vi "Exercise 3.6.vi"(8 "Focal Length":dbl format="%#_g mm", 9 "Groove Density":dbl format="%#_g grooves/mm", 10 "Requested Wavelength (w)":dbl format="%#_g nm", 11 "Slit Width":dbl format="%#_g mm") -> (0 "FWHM":dbl format="%#_g nm", 1 "Min Wavelength":dbl format="%#_g nm", 2 "Max Wavelength":dbl format="%#_g nm", 3 "Linear Dispersion":dbl format="%#_g nm/mm")   [LabVIEW 2020]
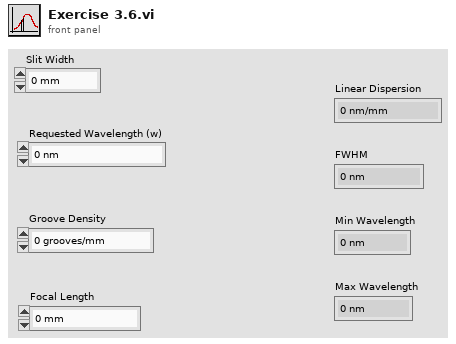
[diagram p1: front panel]
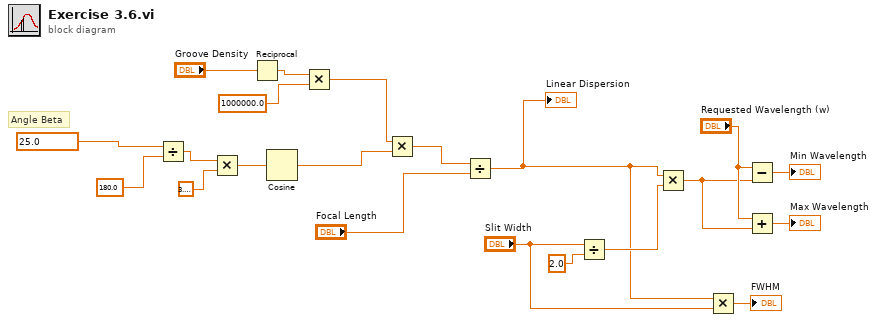
[diagram p0: block diagram]
diagram:
  # "Angle Beta"
  n1 = Divide(x=25.0 ("Diffraction Angle"), y=180.0 ("x")) -> (x/y=w20:dbl)
  n2 = Multiply(x=w20, y=3.141592653589793) -> (x*y=w18:dbl)
  n3 = Reciprocal(x="Groove Density") -> (1/x=w12:dbl)
  n4 = Cosine(x=w18) -> (cos(x)=w21:dbl)
  n5 = Multiply(x=w12, y=1000000.0) -> (x*y=w10:dbl)
  n6 = Multiply(x=w10, y=w21) -> (x*y=w17:dbl)
  n7 = Divide(x=w17, y="Focal Length") -> (x/y=w1:dbl)
  "Linear Dispersion" <- w1
  n8 = Divide(x="Slit Width", y=2.0) -> (x/y=w8:dbl)
  n9 = Multiply(x=w1, y=w8) -> (x*y=w4:dbl)
  n10 = Multiply(x=w1, y="Slit Width") -> (x*y=→"FWHM":dbl)
  n11 = Subtract(x="Requested Wavelength (w)", y=w4) -> (x-y=→"Min Wavelength":dbl)
  n12 = Add(x="Requested Wavelength (w)", y=w4) -> (x+y=→"Max Wavelength":dbl)
